vi "Create All Message Queues.vi"(8 "error in (no error)":errorcluster) -> (0 "error out":errorcluster, 3 "Message Queues out":T1)   [LabVIEW 2018, in "Message Queue.lvlib"]
doc: "This VI creates and initializes all the message queues for your application. If your application requires more than one message queue, right-click the \"Message Queues\" constant above and select Open Type Def. Add the new Message Queue(s) to the type definition, then initialize them in this VI."
uses:
  Message Queue.lvlib
  All Message Queues.ctl
  Message Cluster.ctl
  Enqueue Message (Single).vi
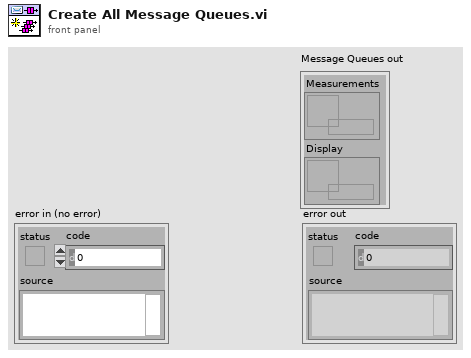
[diagram p1: front panel]
types:
  T1 = typedef "Message Queue.lvlib/All Message Queues.ctl" = cluster{"Measurements":refnum<queue>, "Display":refnum<queue>}
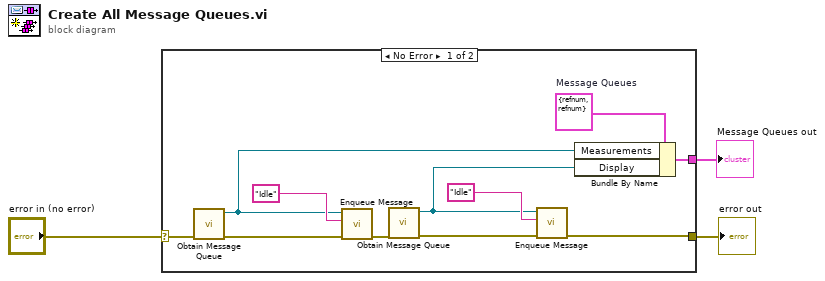
[diagram p0: block diagram]
diagram:
  n1 = case shown="No Error" "error in (no error)" {
    selector: "error in (no error)" -> [w12 w15]
    tunnel: [w4 w15] -> w3
    tunnel: [w13 _] -> w2
    frame No Error {
      w14 = T1 {"Measurements"=refnum, "Display"=refnum}  # Message Queues
      n2 = call "Obtain Message Queue.vi"("error in (no error)"=w12) -> ("error out"=w11:errorcluster, "Message Queue"=w9:refnum<queue>)  [unwired: 9 in]
      n3 = call-poly "Enqueue Message.vi"("error in (no error)"=w11, "Message"="Idle", "Message Queue"=w9) -> ("error out"=w6:errorcluster)  [unwired: 7 in, 1 out]
      n4 = call "Obtain Message Queue.vi"("error in (no error)"=w6) -> ("error out"=w5:errorcluster, "Message Queue"=w7:refnum<queue>)  [unwired: 9 in]
      n5 = call-poly "Enqueue Message.vi"("error in (no error)"=w5, "Message"="Idle", "Message Queue"=w7) -> ("error out"=w4:errorcluster)  [unwired: 7 in, 1 out]
      n6 = Bundle By Name(cluster=w14, "Measurements"=w9, "Display"=w7) -> (w13:T1)
    }
    frame Error {
    }
  }
  "Message Queues out" <- w2
  "error out" <- w3
